vi "Notch (Host).vi"() -> ()   [LabVIEW 2023]
uses:
  <vilib>/rvi/interface/nirviOpenFPGA/nirviOpenFPGA.xnode
  <vilib>/rvi/interface/nirviMethod/nirviMethod.xnode
  <vilib>/rvi/interface/nirviCloseFPGA/nirviCloseFPGA.xnode
  <vilib>/addons/Digital Filter Design/NI_DigFilterLicensed.lvlib
  <vilib>/addons/Digital Filter Design/FXPSim.llb/DFD FXP Postprocessing (I16, nCh).vi
  <vilib>/addons/Digital Filter Design/FilterLib.llb/DFD Load Filter from File.vi
  <vilib>/rvi/errors/niLvFpgaMergeErrorWithErrorCode.vi
  FPGA Bitfiles/Notch_DFDTFilterTarget_Notch(FPGA)_VOQFiOyZLH8.lvbitx
  Notch (FPGA).vi
  <vilib>/userdefined/High Color/nirio_resource_hc.ctl
panel:
  in  "Resource Name":T1="RIO0::INSTR"
  in  "stop":bool
  out "Filtered Signal":dbl[][](graph)
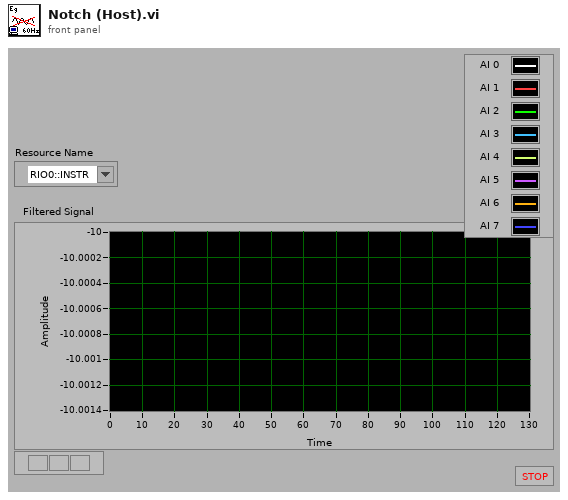
[diagram p1: front panel]
types:
  T1 = typedef "nirio_resource_hc.ctl" = tag
  T2 = typedef "NI_DigFilterLicensed.lvlib/DFD Filter Obj.ctl" = cluster{"mSRate_Fs":dbl, "mSRate_Version":string, "mSRate_Comments":string, "mSRate_OrgCoef":T3, "mSRate_CurCoef":T3, "mSRate_Quantized?":bool, "mSRate_QCoef":T3, "mSRate_QSettings":T5[], "mSRate_Order":i32, "mSRate_Scaling":cluster{"mSRate_ScaleByPowerOf2?":bool, "mSRate_ScaleType":T7}}
  T3 = typedef "NI_DigFilterLicensed.lvlib/DFD Filter Coef.ctl" = cluster{"type":T4, "gain":dbl, "coef a (k)":dbl[], "coef b (v)":dbl[]}
  T4 = typedef "NI_DigFilterLicensed.lvlib/DFD Filter Structure Type Selector.ctl" = enum16{"Undefined", "FIR Direct Form", "FIR Direct Form Transposed", "FIR Symmetric", "FIR Antisymmetric", "IIR Direct Form I", "IIR Direct Form I Transposed", "IIR Direct Form II", "IIR Direct Form II Transposed", "IIR Cascaded Second Order Sections Form I", "IIR Cascaded Second Order Sections Form I Transposed", "IIR Cascaded Second Order Sections Form II", "IIR Cascaded Second Order Sections Form II Transposed", "Lattice Allpass (basic sections)", "Lattice Allpass (one multiplier sections)", "Lattice Allpass (normalized sections)", "Lattice AR (basic sections)", "Lattice AR (one multiplier sections)", "Lattice AR (normalized sections)", "Lattice MA (minimum phase)", "Lattice MA (maximum phase)", "Lattice ARMA (basic sections)", "Lattice ARMA (one multiplier sections)", "Lattice ARMA (normalized sections)"}
  T5 = typedef "NI_DigFilterLicensed.lvlib/dfd_Internal Quantization Settings.ctl" = cluster{"source":T6, "wl":i16, "iwl":i16, "overflow mode":enum16{"Saturation", "Wrap"}, "rounding mode":enum16{"Nearest", "Truncation"}, "signed?":bool}
  T6 = typedef "NI_DigFilterLicensed.lvlib/dfd_Internal Quantization Srcs.ctl" = u16
  T7 = typedef "NI_DigFilterLicensed.lvlib/DFD Coef Norm Type.ctl" = enum16{"No Norm", "Time Domain 1-Norm", "Time Domain 2-Norm", "Time Domain Inf-Norm"}
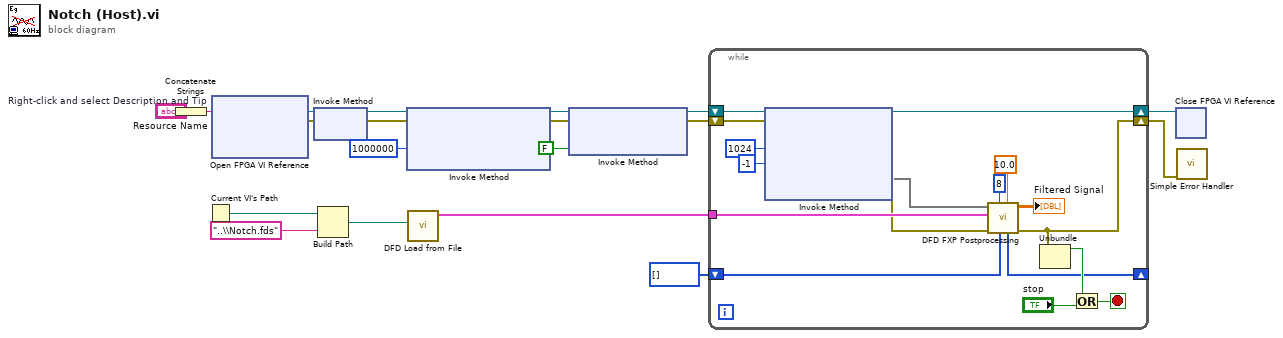
[diagram p0: block diagram]
diagram:
  n1 = Concatenate Strings "Right-click and select Description and Tip"("Resource Name") -> (w1:string)
  n2 = Current VI's Path() -> (path=w6:path)
  n3 = xnode "Open FPGA VI Reference"("resource name"=w1) -> ("FPGA VI Reference Out"=w19:refnum<k20>, "error out"=w18:errorcluster)  [unwired: 1 in]
  n4 = xnode "Invoke Method"("FPGA VI Reference In"=w19, "error in"=w18) -> ("FPGA VI Reference Out"=w17:refnum<k20>, "error out"=w16:errorcluster)
  n5 = Build Path(base path=w6, name or relative path="..\\Notch.fds") -> (appended path=w4:path)
  n6 = xnode "Invoke Method"("FPGA VI Reference In"=w17, "error in"=w16, "Requested Depth"=u32 1000000 ("Depth")) -> ("FPGA VI Reference Out"=w14:refnum<k20>, "error out"=w13:errorcluster)  [unwired: 1 out]
  n7 = call-poly <vilib>:"DFD Load from File.vi"("file path in"=w4) -> ("filter out"=w3:T2)  [unwired: 1 in, 9 out]
  n8 = xnode "Invoke Method"("FPGA VI Reference In"=w14, "error in"=w13, "Wait Until Done (F)"=FALSE) -> ("FPGA VI Reference Out"=w12:refnum<k20>, "error out"=w11:errorcluster)
  n9 = while {
    shift-right: [w27] -> w9
    shift-left: w11 -> [w35]
    tunnel: w3 -> [w32]
    shift-right: [w28] -> w10
    shift-left: w12 -> [w36]
    shift-right: [w22] -> _
    shift-left: i16[] [] ("history out") -> [w21]
    stop <- w24 stop-if-true
    n10 = xnode "Invoke Method"("FPGA VI Reference In"=w36, "error in"=w35, "Number of Elements"=u32 1024, "Timeout (ms)"=-1) -> ("FPGA VI Reference Out"=w28:refnum<k20>, "error out"=w31:errorcluster, "Data"=w20:void[])  [unwired: 1 out]
    n11 = call-poly <vilib>:"DFD FXP Postprocessing.vi"("input range"=10.0, "history in"=w21, "# channels"=8, "error in (no error)"=w31, "filter"=w32, "signal in"=w20) -> ("error out"=w27:errorcluster, "signal out"=→"Filtered Signal":dbl[][], "history out"=w22:i16[])  [unwired: 3 out]
    n12 = Unbundle(w27) -> ("status"=w25:bool)  [unwired: 2 out]
    n13 = Or(x=w25, y="stop") -> (x .or. y?=w24:bool)
  }
  n14 = xnode "Close FPGA VI Reference"("FPGA VI Reference In"=w10) -> ()  [unwired: 1 in, 1 out]
  n15 = call <vilib>:"Simple Error Handler.vi"("error in (no error)"=w9) -> ()  [unwired: 1 in, 8 out]
